vi "Make VI Directory Standard.vi"() -> ()   [LabVIEW 2010]
panel:
  out "Slide":i32(slide) scale=0.0..11.0
  out "filenames":path[](array[path])
  in  "error in":errorcluster
  out "Label Count":i32=-1
  in  "directory":path=path "C:/ATS Development/Code/MyCalc"
  out "error out":errorcluster
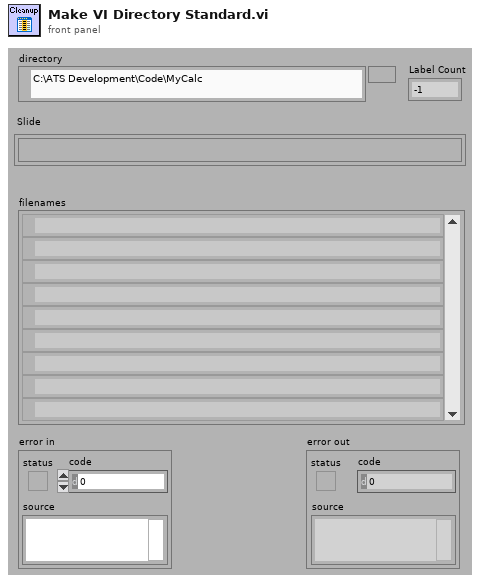
[diagram p1: front panel]
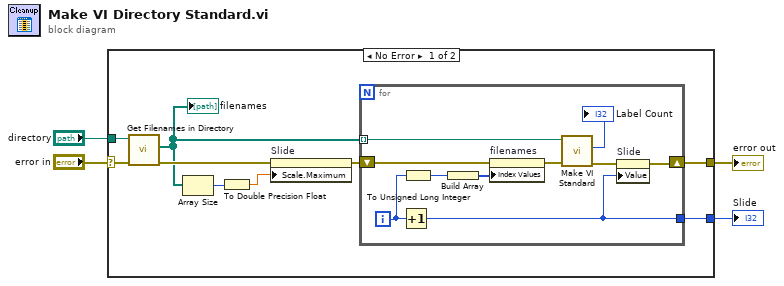
[diagram p0: block diagram]
diagram:
  n1 = case shown="No Error" "error in" {
    selector: "error in" -> [w11 w24]
    tunnel: "directory" -> [w12 _]
    tunnel: [w13 w24] -> w3
    tunnel: [w5 _] -> w1
    frame No Error {
      n2 = call "Get Filenames in Directory.vi"("error in"=w11, "directory path"=w12) -> ("error out"=w10:errorcluster, "filepath array"=w8:path[])  [unwired: 8 in]
      "filenames" <- w8
      n3 = Array Size(array=w8) -> (size(s)=w7:i32)
      n4 = To Double Precision Float(number=w7) -> (double precision float=w6:dbl)
      n5 = property on="Slide" class="Slide (strict)"(error in=w10, "Scale.Maximum"=w6) -> (error out=w9:errorcluster)  [unwired: 1 in, 1 out]
      n6 = for {
        shift-right: [w15] -> w13
        shift-left: w9 -> [w21]
        tunnel: w8 -> [w22] mode=indexing
        tunnel: [w14] -> w5
        i -> [w17]
        n7 = Increment(x=w17) -> (x+1=w14:i32)
        n8 = To Unsigned Long Integer(number=w17) -> (unsigned 32bit integer=w18:u32)
        n9 = Build Array(w18) -> (w19:u32[])
        n10 = property on="filenames" class="Arr (strict)"(error in=w21, "Index Values"=w19) -> (error out=w20:errorcluster)  [unwired: 1 in, 1 out]
        n11 = call "Make VI Standard.vi"("error in"=w20, "vi path"=w22) -> ("error out"=w16:errorcluster, "Label Count"=→"Label Count":i32)  [unwired: 8 in]
        n12 = property on="Slide" class="Slide (strict)"(error in=w16, "Value"=w14) -> (error out=w15:errorcluster)  [unwired: 1 in, 1 out]
      }
    }
    frame Error {
    }
  }
  "error out" <- w3
  "Slide" <- w1
